vi "Filter Lidar Points Outside of Grid.vi"(10 "Encoder-Estimated Absolute Position":cluster{"X":dbl, "Y":dbl}, 11 "Lidar Points":cluster{"X":dbl, "Y":dbl}[](array[cluster])) -> (3 "Filtered lidar points in the grid":cluster{"X":dbl, "Y":dbl}[](array[cluster]))   [LabVIEW 2017]
panel:
  in  "Width of Course (mm)":dbl=500.0 format="%#_13g"
  in  "Lookahead Limit":dbl=2000.0 format="%#_13g"
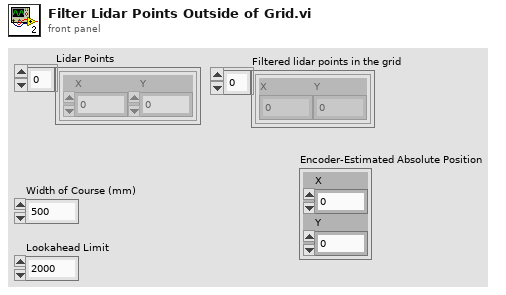
[diagram p1: front panel]
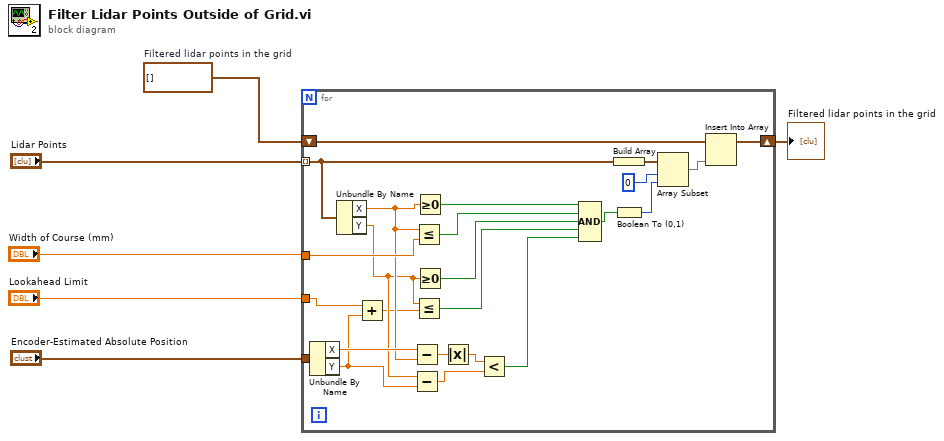
[diagram p0: block diagram]
diagram:
  w2 = cluster{"X":dbl, "Y":dbl}[] []  # Filtered lidar points in the grid
  n1 = for {
    tunnel: "Lidar Points" -> [w24] mode=indexing
    shift-right: [w30] -> w6
    shift-left: w2 -> [w29]
    tunnel: "Width of Course (mm)" -> [w22]
    tunnel: "Lookahead Limit" -> [w8]
    tunnel: "Encoder-Estimated Absolute Position" -> [w17]
    n2 = Unbundle By Name(w17) -> ("X"=w16:dbl, "Y"=w9:dbl)
    n3 = Unbundle By Name(w24) -> ("X"=w15:dbl, "Y"=w12:dbl)
    n4 = Add(x=w8, y=w9) -> (x+y=w7:dbl)
    n5 = Subtract(x=w16, y=w15) -> (x-y=w14:dbl)
    n6 = Subtract(x=w12, y=w9) -> (x-y=w11:dbl)
    n7 = Less Or Equal?(x=w15, y=w22) -> (x <= y?=w21:bool)
    n8 = Less Or Equal?(x=w12, y=w7) -> (x <= y?=w19:bool)
    n9 = Greater Or Equal To 0?(x=w15) -> (x >= 0?=w23:bool)
    n10 = Greater Or Equal To 0?(x=w12) -> (x >= 0?=w20:bool)
    n11 = Absolute Value(x=w14) -> (abs(x)=w13:dbl)
    n12 = Less?(x=w13, y=w11) -> (x < y?=w10:bool)
    n13 = Compound Arithmetic op=AND(w23, w21, w20, w19, w10) -> (w18:bool)
    n14 = Build Array(w24) -> (w28:cluster{"X":dbl, "Y":dbl}[])
    n15 = Boolean To (0,1)(Boolean=w18) -> (0, 1=w25:i16)
    n16 = Array Subset(array=w28, index=0, length=w25) -> (w26:cluster{"X":dbl, "Y":dbl}[])
    n17 = Insert Into Array(array=w29, new element=w26) -> (w30:cluster{"X":dbl, "Y":dbl}[])  [unwired: 1 in]
  }
  "Filtered lidar points in the grid" <- w6
